vi "Init Sim Servo Motor.vi"(8 "error in (no error)":errorcluster, 10 "device ID":T1, 11 "NI_Robotics_Starter Kit Host_Sim_1.0 in":refnum<class "NI_Robotics_Starter Kit Host_Sim_1.0.lvclass">) -> (0 "error out":errorcluster, 3 "NI_Robotics_Starter Kit Host_Sim_1.0 out":refnum<class "NI_Robotics_Starter Kit Host_Sim_1.0.lvclass">)   [LabVIEW 2017, in "NI_Robotics_Starter Kit Host_Sim_1.0.lvclass"]
uses:
  <vilib>/robotics/Starter Kit/1.0/Sim Host Interface/NI_Robotics_Starter Kit Host_Sim_1.0.lvclass
  c:/Program Files (x86)/National Instruments/LabVIEW 2017/vi.lib/robotics/Starter Kit/Host Interface/NI_Robotics_Starter Kit Host.lvclass
  <vilib>/robotics/Simulator/Engine/ctl/DeviceID.ctl
  <vilib>/robotics/Starter Kit/Host Interface/NI_Robotics_Starter Kit Host.lvclass/NI_Robotics_Starter Kit Host.ctl
  <vilib>/robotics/Starter Kit/Servo Motor 1.0/NI_Robotics_Starter Kit Servo Motor_1.0.lvclass
  c:/Program Files (x86)/National Instruments/LabVIEW 2017/vi.lib/robotics/Starter Kit/Servo Motor/NI_Robotics_Starter Kit Servo Motor.lvclass
  <instrlib>/Parallax Standard Servo/HAIOL/Simulator/Parallax Standard Servo Simulator.lvclass
  <vilib>/robotics/Starter Kit/Host Interface/NI_Robotics_Starter Kit Host.lvclass
  <vilib>/robotics/Utilities/NI_Robotics Utilities.lvlib
  <vilib>/robotics/Simulator/NI_Robotics_Simulator.lvlib
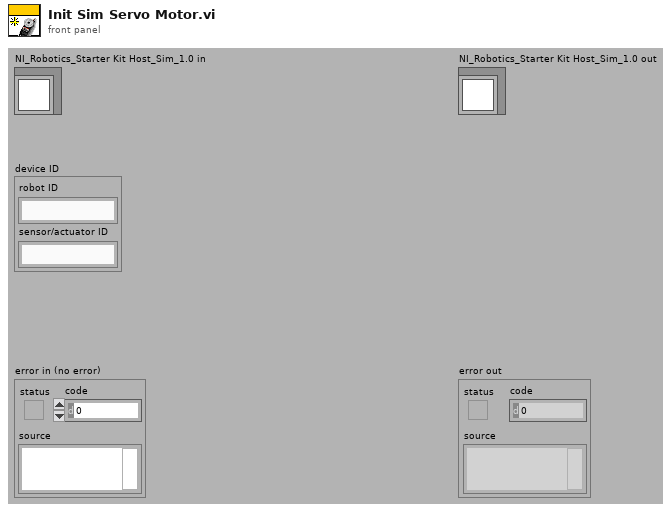
[diagram p1: front panel]
types:
  T1 = typedef "NI_Robotics_Simulator.lvlib/DeviceID.ctl" = cluster{"robot ID":string, "sensor/actuator ID":string}
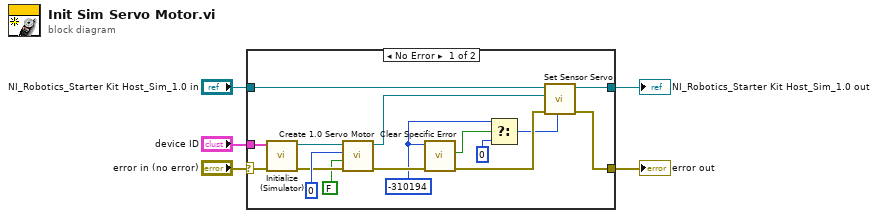
[diagram p0: block diagram]
diagram:
  n1 = case shown="No Error" "error in (no error)" {
    selector: "error in (no error)" -> [w13 w23]
    tunnel: "device ID" -> [w21 _]
    tunnel: "NI_Robotics_Starter Kit Host_Sim_1.0 in" -> [w17 w22]
    tunnel: [w16 w22] -> w3
    tunnel: [w14 w23] -> w2
    frame No Error {
      w7 = -310194 ("code")
      n2 = call <instrlib>:"Initialize (Simulator).vi"("error in (no error)"=w13, "Device ID"=w21) -> ("error out"=w18:errorcluster, "Parallax Standard Servo out"=w20:refnum<class "Parallax Standard Servo.lvclass">)  [unwired: 8 in]
      n3 = call <vilib>:"Create 1.0 Servo Motor.vi"("error in (no error)"=w18, "apply offset angle from file (T)"=FALSE, "servo ID"=0, "Parallax standard servo"=w20) -> ("error out"=w11:errorcluster, "Starter Kit Servo Motor_1.0 out"=w15:refnum<class "NI_Robotics_Starter Kit Servo Motor_1.0.lvclass">)  [unwired: 6 in]
      n4 = call <vilib>:"Clear Specific Error.vi"("error in (no error)"=w11, "code"=w7) -> ("error out"=w10:errorcluster, "cleared?"=w8:bool)  [unwired: 7 in, 1 out]
      n5 = Select(t=w7, s=w8, f=0) -> (s? t:f=w6:i32)
      n6 = call <vilib>:"Set Sensor Servo.vi"("sensor servo error (0)"=w6, "error in (no error)"=w10, "sensor servo"=w15, "NI_Robotics_Starter Kit Host in"=w17) -> ("error out"=w14:errorcluster, "NI_Robotics_Starter Kit Host out"=w16:refnum<class "NI_Robotics_Starter Kit Host_Sim_1.0.lvclass">)  [unwired: 6 in]
    }
    frame Error {
    }
  }
  "error out" <- w2
  "NI_Robotics_Starter Kit Host_Sim_1.0 out" <- w3
